vi "SensorHEX2Name.vi"(11 "Sensor HEX":u8 format="%x") -> (3 "Sensor name":string)   [LabVIEW 2018]
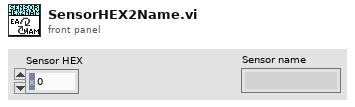
[diagram p1: front panel]
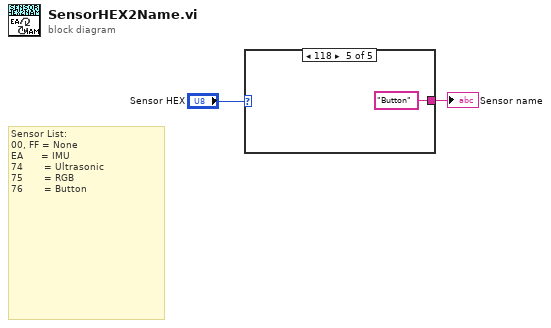
[diagram p0: block diagram]
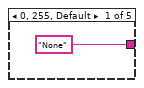
[diagram p2: hidden frame]
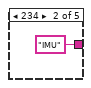
[diagram p3: hidden frame]
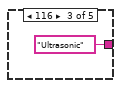
[diagram p4: hidden frame]
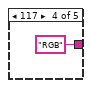
[diagram p5: hidden frame]
diagram:
  # "Sensor List:\n00, FF = None\nEA      = IMU\n74       = Ultrasonic\n75       = RGB\n76       = Button"
  n1 = case shown="118" "Sensor HEX" {
    tunnel: ["None" "IMU" "Ultrasonic" "RGB" "Button"] -> w1
    frame 0, 255, Default {
    }
    frame 234 {
    }
    frame 116 {
    }
    frame 117 {
    }
    frame 118 {
    }
  }
  "Sensor name" <- w1
